vi "Initialize.vi"(8 "error in (no error)":errorcluster, 11 "Microscope":refnum<class "Microscope.lvclass">) -> (0 "error out":errorcluster, 3 "Microscope out":refnum<class "Microscope.lvclass">)   [LabVIEW 2013, in "Microscope.lvclass"]
doc: "---------------------------------------------------------------\nJKI State Machine Objects™\nhttp://jki.net/state-machine-objects/\nCopyright (C) 2005-2015, JKI <info@jki.net>\nALL RIGHTS RESERVEDJKI State Machine Objects (SMO) 1.0.0.4\nJKI - JKI\nCopyright (c) 2015, JKI"
uses:
  Microscope.lvclass
  Typedefs/PrivateEvents--Microscope.Initialize.ctl
panel:
  # "For instructions on how to use the JKI State Machine Objects, examples and video tutorials, visit:\nhttp://jki.net/state-machine-objects/\n\nJKI State Machine Objects™\nhttp://jki.net/state-machine-objects/\nCopyright (C) 2005-2015, JKI <info@jki.net>\nALL RIGHTS RESERVED"
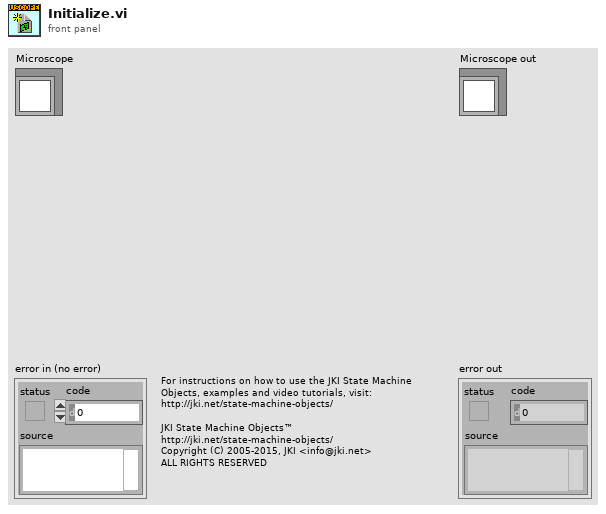
[diagram p1: front panel]
types:
  T1 = typedef "Microscope.lvclass/PrivateEvents--Microscope.Initialize.ctl" = bool
  T2 = typedef "Microscope.lvclass/PrivateEvents--Cluster.ctl" = cluster{"New Value":refnum<user-event>, "Initialize":refnum<user-event>, "CaptureImageAtPosition":refnum<user-event>}
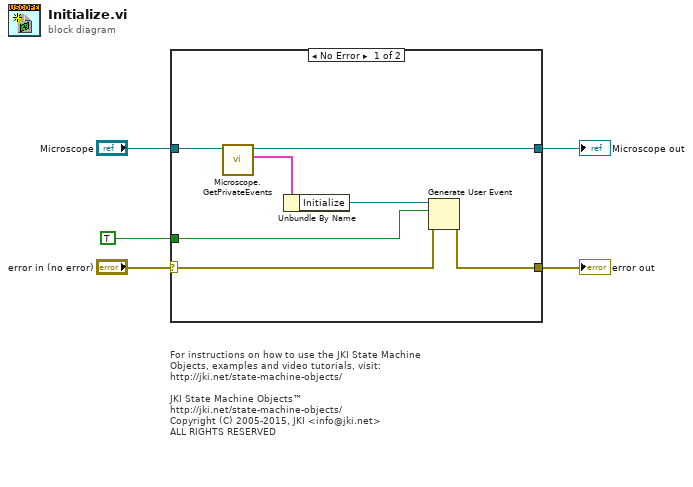
[diagram p0: block diagram]
diagram:
  # "For instructions on how to use the JKI State Machine Objects, examples and video tutorials, visit:\nhttp://jki.net/state-machine-objects/\n\nJKI State Machine Objects™\nhttp://jki.net/state-machine-objects/\nCopyright (C) 2005-2015, JKI <info@jki.net>\nALL RIGHTS RESERVED"
  n1 = case shown="No Error" "error in (no error)" {
    selector: "error in (no error)" -> [w12 w14]
    tunnel: [w8 w14] -> w4
    tunnel: [w6 w13] -> w5
    tunnel: "Microscope" -> [w7 w13]
    tunnel: T1 TRUE ("Initialize") -> [w11 _]
    frame No Error {
      n2 = call "Microscope.GetPrivateEvents.vi"("Microscope"=w7) -> ("Private Events"=w10:T2, "Microscope out"=w6:refnum<class "Microscope.lvclass">)  [unwired: 8 in, 1 out]
      n3 = Unbundle By Name(w10) -> ("Initialize"=w9:refnum<user-event>)
      n4 = Generate User Event(user event=w9, event data cluster=w11, error in=w12) -> (error out=w8:errorcluster)  [unwired: 1 in, 1 out]
    }
    frame Error {
    }
  }
  "error out" <- w4
  "Microscope out" <- w5
